vi "CheckFailItem.vi"(11 "in":string[](array[string])) -> (3 "out":string[](array[string]))   [LabVIEW 2019, in "LocalReport.lvlib" / "LocalReport.lvclass"]
uses:
  LocalReport.lvclass
  e39797e9-d1cd-484f-9c8c-bd2636b9b08e.vi
  c512f17e-c3a6-4030-b767-d66084533eb2.vi
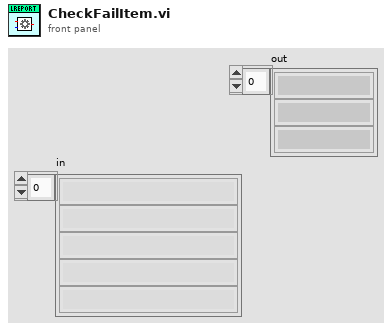
[diagram p1: front panel]
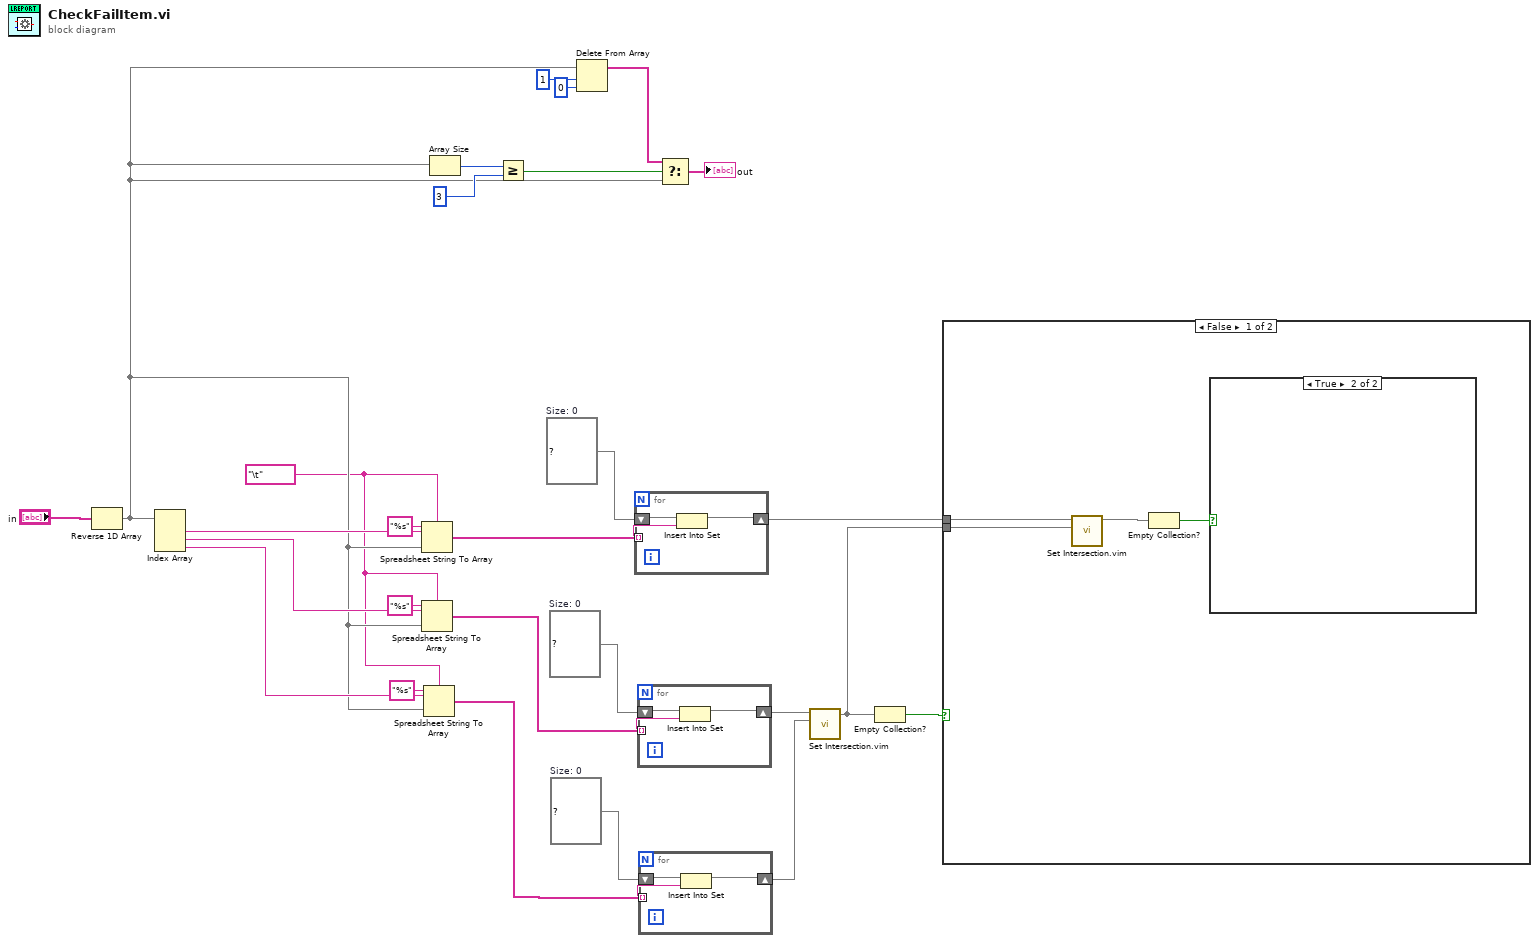
[diagram p0: block diagram]
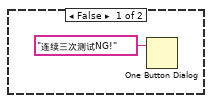
[diagram p2: hidden frame]
diagram:
  w1 = "\t" ("delimiter (Tab)")
  w15 = set{string} {}  # Size: 0
  w17 = set{string} {}  # Size: 0
  w20 = set{string} {}  # Size: 0
  n1 = Reverse 1D Array(array="in") -> (reversed array=w3:string[])
  n2 = Index Array(array=w3) -> (element #1=w26:string, element #2=w24:string, element #3=w22:string)  [unwired: 3 in]
  n3 = Spreadsheet String To Array(delimiter (Tab)=w1, format string="%s" ("格式字符串"), spreadsheet string=w26, array type (2D Dbl)=w3) -> (array=w21:string[])
  n4 = Spreadsheet String To Array(delimiter (Tab)=w1, format string="%s" ("格式字符串"), spreadsheet string=w24, array type (2D Dbl)=w3) -> (array=w16:string[])
  n5 = Spreadsheet String To Array(delimiter (Tab)=w1, format string="%s" ("格式字符串"), spreadsheet string=w22, array type (2D Dbl)=w3) -> (array=w14:string[])
  n6 = Array Size(array=w3) -> (size(s)=w9:i32)
  n7 = Greater Or Equal?(x=w9, y=3) -> (x >= y?=w7:bool)
  n8 = Delete From Array(array=w3, length=1 ("长度"), index=0 ("索引")) -> (array with subset deleted=w4:string[])  [unwired: 1 out]
  n9 = for {
    tunnel: w21 -> [w28] mode=indexing
    shift-right: [w30] -> w19
    shift-left: w20 -> [w29]
    n10 = Insert Into Set(10:w28, 11:w29) -> (3:w30:set{string})  [unwired: 1 out]
  }
  n11 = for {
    tunnel: w16 -> [w31] mode=indexing
    shift-right: [w33] -> w18
    shift-left: w17 -> [w32]
    n12 = Insert Into Set(10:w31, 11:w32) -> (3:w33:set{string})  [unwired: 1 out]
  }
  n13 = for {
    tunnel: w14 -> [w34] mode=indexing
    shift-right: [w36] -> w13
    shift-left: w15 -> [w35]
    n14 = Insert Into Set(10:w34, 11:w35) -> (3:w36:set{string})  [unwired: 1 out]
  }
  n15 = Select(t=w4, s=w7, f=w3) -> (s? t:f=→"out":string[])
  n16 = call "Set Intersection.vim"("set 2"=w13, "set 1"=w18) -> ("intersection"=w11:set{string})  [unwired: 9 in]
  n17 = Empty Collection?(1:w11) -> (0:w12:bool)
  n18 = case shown="False" w12 {
    tunnel: w19 -> [w40 _]
    tunnel: w11 -> [w39 _]
    frame False {
      n19 = call "Set Intersection.vim"("set 2"=w39, "set 1"=w40) -> ("intersection"=w38:set{string})  [unwired: 9 in]
      n20 = Empty Collection?(1:w38) -> (0:w37:bool)
      n21 = case shown="True" w37 {
        frame False {
          n22 = One Button Dialog(message="连续三次测试NG!" ("消息")) -> ()  [unwired: 1 in, 1 out]
        }
        frame True {
        }
      }
    }
    frame True {
    }
  }
